vi "thinned_image_to_centerline_debug.vi"() -> ()   [LabVIEW 2019]
uses:
  StimulusObject.lvclass
  iterative_thinned_image_to_segment.vi
  pixel_XY_to_1D_index.vi
  thinned_image_to_centerline.vi/a49f2ef7-d53c-4424-bee3-5857753b5dab.vi
  iterative_segments_to_centerline.vi
  1D_index_to_pixel_XY.vi
  iterative_segments_to_centerline_oneiteration.vi
  <vilib>/vision/NI_Vision_Development_Module.lvlib
panel:
  out "error out":errorcluster
  out "Original Image":T1(plugin-control)
  out "Algorithm timed out":bool
  out "Centerline":i32[][](array[numeric])
  out "Acquired Image":T1(plugin-control)
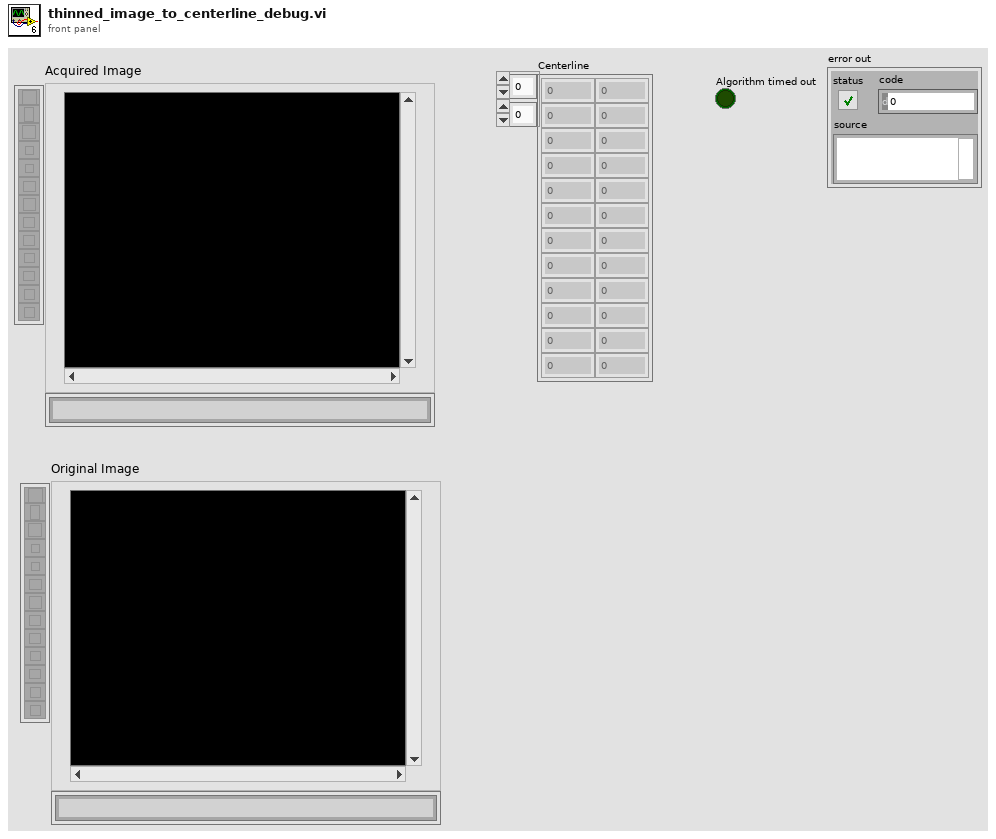
[diagram p1: front panel]
types:
  T1 = typedef "IMAQ Image.ctl" = refnum<image>
  T2 = typedef "Image Type" = u32
  T3 = typedef "Particle Parameters" = i32
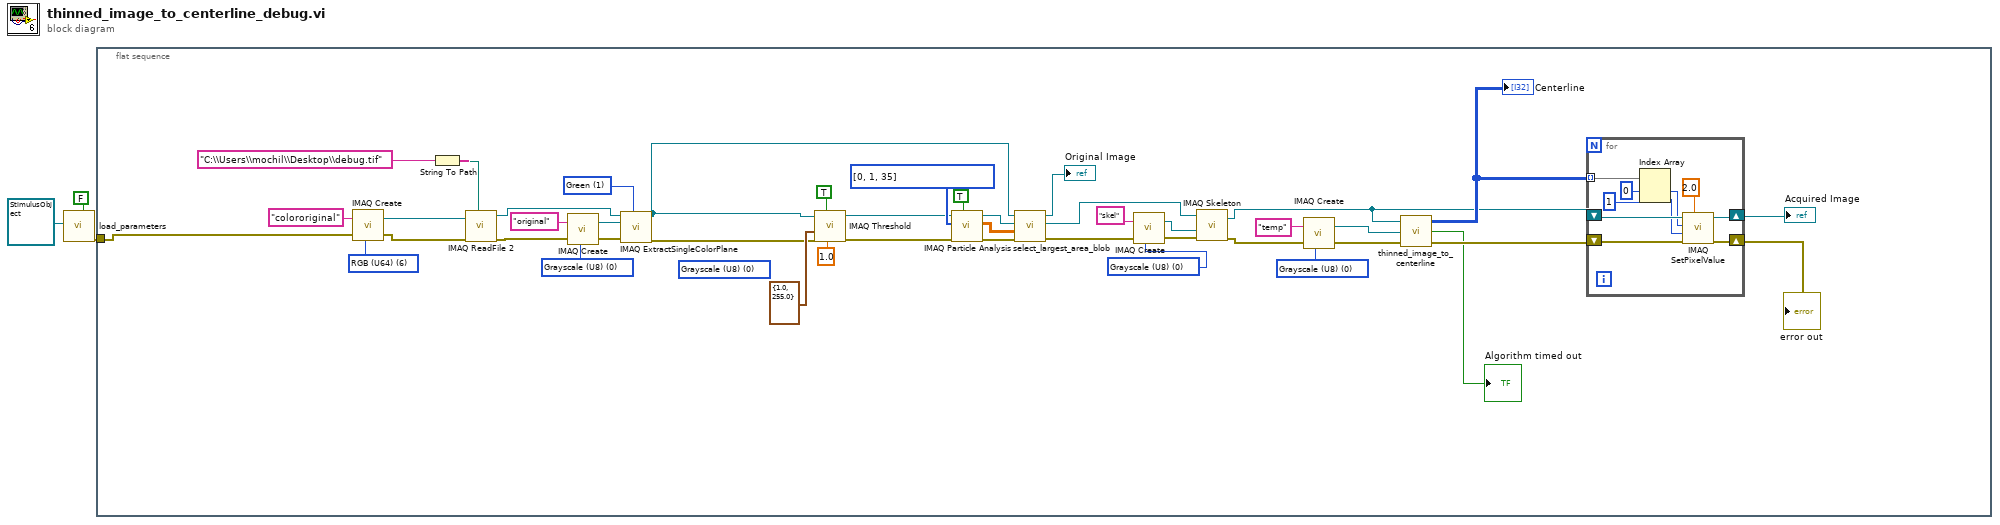
[diagram p0: block diagram]
diagram:
  n1 = call "load_parameters.vi"("Set Up Projector and Camera (T)"=FALSE ("Full Setup"), "StimulusObjectClassInput"=refnum<class "StimulusObject.lvclass"> refnum) -> ("error out"=w3:errorcluster)  [unwired: 7 in, 2 out]
  n2 = flat-sequence {
    tunnel: w3 -> [w14]
    frame #0 {
      w7 = 1 items=["Red", "Green", "Blue", "Hue", "Saturation", "Luminance", "Value", "Intensity"] ("Color Plane")
      w15 = T2 6 items=["Grayscale (U8)", "Grayscale (I16)", "Grayscale (SGL)", "Complex (CSG)", "RGB (U32)", "HSL (U32)", "RGB (U64)", "Grayscale (U16)"] ("Image Type")
      w17 = T2 0 items=["Grayscale (U8)", "Grayscale (I16)", "Grayscale (SGL)", "Complex (CSG)", "RGB (U32)", "HSL (U32)", "RGB (U64)", "Grayscale (U16)"] ("Image Type")
      w29 = T3[] [0, 1, 35] items=["Center of Mass X", "Center of Mass Y", "First Pixel X", "First Pixel Y", "Bounding Rect Left", "Bounding Rect Top", "Bounding Rect Right", "Bounding Rect Bottom", "Max Feret Diameter Start X", "Max Feret Diameter Start Y", "Max Feret Diameter End X", "Max Feret Diameter End Y", "Max Horiz. Segment Length Left", "Max Horiz. Segment Length Right", "Max Horiz. Segment Length Row", "-", "Bounding Rect Width", "Bounding Rect Height", "Bounding Rect Diagonal", "Perimeter", "Convex Hull Perimeter", "Holes' Perimeter", "Max Feret Diameter", "Equivalent Ellipse Major Axis", "Equivalent Ellipse Minor Axis", "Equivalent Ellipse Minor Axis (Feret)", "Equivalent Rect Long Side", "Equivalent Rect Short Side", "Equivalent Rect Diagonal", "Equivalent Rect Short Side (Feret)", "Average Horiz. Segment Length", "Average Vert. Segment Length", "Hydraulic Radius", "Waddel Disk Diameter", "-", "Area", "Holes' Area", "Particle & Holes' Area", "Convex Hull Area", "Image Area", "-", "Number of Holes", "Number of Horiz. Segments", "Number of Vert. Segments", "-", "Orientation", "Max Feret Diameter Orientation", "-", "% Area/Image Area", "% Area/(Particle & Holes' Area)", "Ratio of Equivalent Ellipse Axes", "Ratio of Equivalent Rect Sides", "-", "Elongation Factor", "Compactness Factor", "Heywood Circularity Factor", "Type Factor", "-", "Sum X", "Sum Y", "Sum XX", "Sum XY", "Sum YY", "Sum XXX", "Sum XXY", "Sum XYY", "Sum YYY", "-", "Moment of Inertia XX", "Moment of Inertia XY", "Moment of Inertia YY", "Moment of Inertia XXX", "Moment of Inertia XXY", "Moment of Inertia XYY", "Moment of Inertia YYY", "Norm. Moment of Inertia XX", "Norm. Moment of Inertia XY", "Norm. Moment of Inertia YY", "Norm. Moment of Inertia XXX", "Norm. Moment of Inertia XXY", "Norm. Moment of Inertia XYY", "Norm. Moment of Inertia YYY", "Hu Moment 1", "Hu Moment 2", "Hu Moment 3", "Hu Moment 4", "Hu Moment 5", "Hu Moment 6", "Hu Moment 7"] ("Pixel Measurements")
      w4 = T2 0 items=["Grayscale (U8)", "Grayscale (I16)", "Grayscale (SGL)", "Complex (CSG)", "RGB (U32)", "HSL (U32)", "RGB (U64)", "Grayscale (U16)"] ("Image Type")
      (unwired) T2 0 items=["Grayscale (U8)", "Grayscale (I16)", "Grayscale (SGL)", "Complex (CSG)", "RGB (U32)", "HSL (U32)", "RGB (U64)", "Grayscale (U16)"] ("Image Type")
      w41 = T2 0 items=["Grayscale (U8)", "Grayscale (I16)", "Grayscale (SGL)", "Complex (CSG)", "RGB (U32)", "HSL (U32)", "RGB (U64)", "Grayscale (U16)"] ("Image Type")
      n3 = call "IMAQ Create"("Image Name"="colororiginal", "Image Type"=w15, "error in (no error)"=w14) -> ("New Image"=w11:T1, "error out"=w13:errorcluster)  [unwired: 2 in]
      n4 = String To Path(string="C:\\Users\\mochil\\Desktop\\debug.tif") -> (path=w46:path)
      n5 = call "IMAQ ReadFile 2"("File Path"=w46, "error in (no error)"=w13, "Image"=w11) -> ("error out"=w12:errorcluster, "Image Out"=w8:T1)  [unwired: 4 in, 3 out]
      n6 = call "IMAQ Create"("Image Name"="original", "Image Type"=w17, "error in (no error)"=w12) -> ("New Image"=w9:T1, "error out"=w10:errorcluster)  [unwired: 2 in]
      n7 = call "IMAQ ExtractSingleColorPlane"("Color Plane"=w7, "error in (no error)"=w10, "Image Dst"=w9, "Image Src"=w8) -> ("error out"=w6:errorcluster, "Image Dst Out"=w5:T1)  [unwired: 6 in]
      n8 = call "IMAQ Threshold"("Replace Value"=sgl 1.0, "Keep/Replace Value (Replace)"=TRUE, "error in (no error)"=w6, "Range"=cluster{"Lower value":sgl, "Upper value":sgl} {"Lower value"=1.0, "Upper value"=255.0}, "Image Src"=w5) -> ("error out"=w25:errorcluster, "Image Dst Out"=w22:T1)  [unwired: 5 in]
      n9 = call "IMAQ Particle Analysis"("Connectivity 4/8 (8)"=TRUE, "error in (no error)"=w25, "Pixel Measurements"=w29, "Image"=w22) -> ("error out"=w26:errorcluster, "Particle Measurements (Pixels)"=w27:dbl[][], "Image Out (duplicate)"=w21:T1)  [unwired: 2 in, 3 out]
      n10 = call "select_largest_area_blob.vi"("error in (no error)"=w26, "Particle Measurements (Pixels) In"=w27, "Binary Image In"=w21, "Original Image In"=w5) -> ("error out"=w24:errorcluster, "Binary Image Out"=w23:T1, "Original Image Out"=→"Original Image":T1)  [unwired: 1 out]
      n11 = call "IMAQ Create"("Image Name"="skel", "Image Type"=w4, "error in (no error)"=w24) -> ("New Image"=w30:T1, "error out"=w31:errorcluster)  [unwired: 2 in]
      n12 = call "IMAQ Skeleton"("error in (no error)"=w31, "Image Dst"=w30, "Image Src"=w23) -> ("error out"=w35:errorcluster, "Image Dst Out"=w36:T1)  [unwired: 3 in]
      n13 = call "IMAQ Create"("Image Name"="temp", "Image Type"=w41, "error in (no error)"=w35) -> ("New Image"=w43:T1, "error out"=w42:errorcluster)  [unwired: 2 in]
      n14 = call "thinned_image_to_centerline.vi"("error in"=w42, "Temp Image"=w43, "Skeleton Image"=w36) -> ("error out"=w45:errorcluster, "Algorithm timed out"=→"Algorithm timed out":bool, "Centline Pixels"=w37:i32[][])
      "Centerline" <- w37
      n15 = for {
        tunnel: w37 -> [w55] mode=indexing
        shift-right: [w49] -> w34
        shift-left: w36 -> [w57]
        shift-right: [w48] -> w19
        shift-left: w45 -> [w56]
        n16 = Index Array(array=w55, index #1=0 ("index"), index #2=1 ("index")) -> (element #1=w52:i32, element #2=w51:i32)
        n17 = call "IMAQ SetPixelValue"("Pixel Value"=sgl 2.0, "error in (no error)"=w56, "Y Coordinate"=w51, "X Coordinate"=w52, "Image"=w57) -> ("error out"=w48:errorcluster, "Image Out"=w49:T1)  [unwired: 5 in]
      }
      "Acquired Image" <- w34
      "error out" <- w19
    }
  }
